vi "Prefix.vi"(10 "Prefix to Add to Label":string) -> (3 "Translator":refnum<class "LabelPrefix.lvclass">)   [LabVIEW 2011, in "Messenging.lvlib" / "LabelPrefix.lvclass"]
uses:
  LabelPrefix.lvclass
  LabelPrefix.lvclass/LabelPrefix.ctl
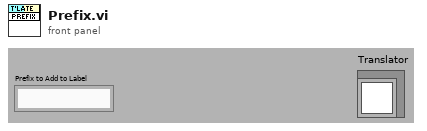
[diagram p1: front panel]
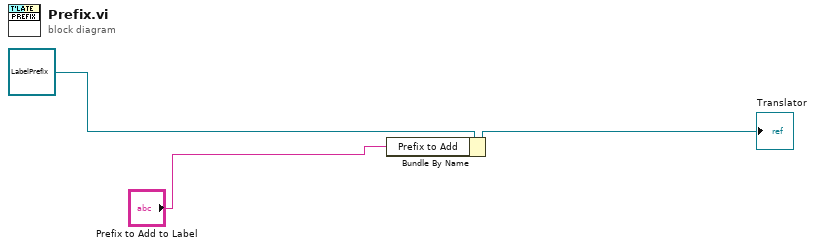
[diagram p0: block diagram]
diagram:
  n1 = Bundle By Name(cluster=refnum<class "LabelPrefix.lvclass"> refnum ("SubstututeMessage in"), "Prefix to Add"="Prefix to Add to Label") -> (→"Translator":refnum<class "LabelPrefix.lvclass">)
